vi "Square Inputs.vi"(11 "Input":dbl) -> (3 "Squared Value":dbl)   [LabVIEW 2012]
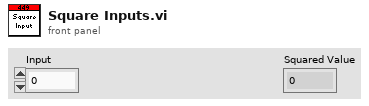
[diagram p1: front panel]
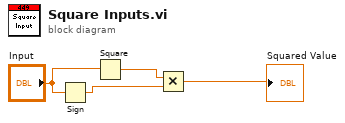
[diagram p0: block diagram]
diagram:
  n1 = Sign(1:"Input") -> (0:w2:dbl)
  n2 = Square(x="Input") -> (x^2=w3:dbl)
  n3 = Multiply(x=w3, y=w2) -> (x*y=→"Squared Value":dbl)
